vi "8bit sync-Populate Codec control.vi"() -> (1 "Codec Names":string[](array[string]))   [LabVIEW 2020]
uses:
  Globals/gl_8-bit montage window ctrl refs.vi
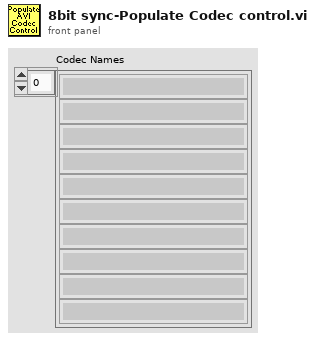
[diagram p1: front panel]
types:
  T1 = typedef "8-bit video export window ctrl refs.ctl" = cluster{"This VI":refnum<vi>, "Add speed data":refnum<vi>, "Add camera videos":refnum<vi>, "Stop button":refnum<vi>, "Camera Video Adjustments":refnum<vi>, "Microscope Image Adjustments":refnum<vi>, "Execute":refnum<vi>, "Codec":refnum<vi>, "Channel to load":refnum<vi>, "Speed graph behaviour":refnum<vi>, "Include speed graph":refnum<vi>, "Number of rows to generate":refnum<vi>, "Path":refnum<vi>}
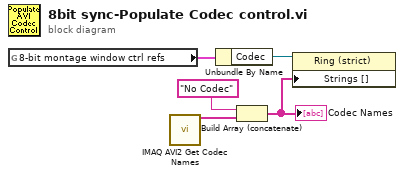
[diagram p0: block diagram]
diagram:
  n1 = global read "gl_8-bit montage window ctrl refs.vi" "8-bit montage window ctrl refs"() -> (w3:T1)
  n2 = call "IMAQ AVI2 Get Codec Names"() -> ("Codec Names"=w5:string[])  [unwired: 10 in, 1 out]
  n3 = Unbundle By Name(w3) -> ("Codec"=w2:refnum<vi>)
  n4 = Build Array (concatenate)("No Codec" ("Codec Name"), w5) -> (w1:string[])
  "Codec Names" <- w1
  n5 = property class="Ring (strict)"(reference=w2, "Strings []"=w1) -> ()  [unwired: 1 in, 2 out]
